vi "Main.vi"() -> ()   [LabVIEW 2017]
uses:
  CTL/REF Channel Select.ctl
  D:/test/PDLSTS/LV_PDL_Sample/DLL/STSProcess.dll
  DLL/STSProcess.dll
  CTL/Address Cluster.ctl
  D:/test/PDLSTS/LV_PDL_Sample/DLL/InstrumentDLL.dll
  DLL/InstrumentDLL.dll
  <vilib>/Utility/miscctls.llb/LVStringsAndValuesArrayTypeDef_DBL.ctl
panel:
  in  "btnsavecalil":bool
  in  "txtsaverange":i32=1 caption="Range"
  in  "chksavemu":bool
  in  "chk2scan":bool
  in  "PDLSTS":refnum<k24>
  in  "btnzeroing":bool
  in  "btnreadref_data":bool
  in  "btnsaveRawdata":bool
  in  "btnsaveref_rawdata":bool
  in  "chkeach_ch":bool
  in  "btnmeas":bool
  in  "btnset":bool
  in  "Range1":bool
  in  "REF Channel Select":T1={"M1S0C1"=TRUE, "M1S0C2"=FALSE, "M1S0C3"=FALSE, "M1S0C4"=FALSE, "M1S1C1"=FALSE, "M1S1C2"=FALSE, "M1S1C3"=FALSE, "M1S1C4"=FALSE, "M1S2C1"=FALSE, "M1S2C2"=FALSE, "M1S2C3"=FALSE, "M1S2C4"=FALSE, "M1S3C1"=FALSE, "M1S3C2"=FALSE, "M1S3C3"=FALSE, "M1S3C4"=FALSE, "M1S4C1"=FALSE, "M1S4C2"=FALSE, "M1S4C3"=FALSE, "M1S4C4"=FALSE, "M2S0C1"=FALSE, "M2S0C2"=FALSE, "M2S0C3"=FALSE, "M2S0C4"=FALSE, "M2S1C1"=FALSE, "M2S1C2"=FALSE, "M2S1C3"=FALSE, "M2S1C4"=FALSE, "M2S2C1"=FALSE, "M2S2C2"=FALSE, "M2S2C3"=FALSE, "M2S2C4"=FALSE, "M2S3C1"=FALSE, "M2S3C2"=FALSE, "M2S3C3"=FALSE, "M2S3C4"=FALSE, "M2S4C1"=FALSE, "M2S4C2"=FALSE, "M2S4C3"=FALSE, "M2S4C4"=FALSE}
  in  "Range2":bool
  in  "Range3":bool
  in  "Range4":bool
  in  "Range5":bool
  in  "btnget_reference":bool
  in  "Address Cluster":T2={"SPU"=refnum, "MPM"=[], "Port_Count"=0.0, "MPM_Count"=0.0, "SPU_Resource"=[], "USB_Resource"=[], "MPM_Communicater"="", "MPM_Count"=0.0, "MPM_Address"=[], "MPM_Portnumber"=[], "SPU_DeviveID"="", "MPM_communcation_method"=[], "TSL_sweepstartwave"=0.0, "TSL_sweepstopwave"=0.0, "TSL_Address"="", "TSL_Communicater"="", "TSL"=refnum, "tsl_communcation_method"=3, "TSL_Portnumber"=0.0, "PCU"=refnum, "PCU_Communicater"="", "PCU_Address"="", "PCU_Portnumber"=0.0, "PCU_useing_internal_DAQ"=FALSE, "PCU_communcation_method"=0} {"PCU_communcation_method" items=["GPIB", "C232C", "TCPIP", "USB"]; "tsl_communcation_method" items=["GPIB", "C232C", "TCPIP", "USB"]; "MPM_communcation_method" items=["GPIB", "C232C", "TCPIP", "USB"]}
  in  "Active Sensors":bool[](array[boolean])
  out "Meas_rang":i32[](array[numeric])
  out "Flag_213":bool
  out "Flag_215":bool
  out "Mergedata_struct":refnum<k24>[](array[refnum])
  out "Meas_monitor_struct":refnum<k24>[](array[refnum])
  out "Ref_monitordata_struct":refnum<k24>[](array[refnum])
  out "Refdata_struct":refnum<k24>[](array[refnum])
  out "Data_struct":refnum<k24>[](array[refnum])
  in  "txtpower":dbl caption="TSL Power(dBm)"
  in  "cmbspeed":u16(ring) caption="SweepSpeed(nm/sec)" items=["1"=1, "5"=5, "10"=10, "20"=20, "40"=40, "50"=50, "80"=80, "100"=100]
  in  "txtstepwave":dbl=0.01 caption="WavelengthStep(nm)"
  in  "txtstopwave":dbl caption="StopWavelength(nm)"
  in  "txtstartwave":dbl caption="StartWavelength(nm)"
  # "Measurement ch"
  # "Measurement Range"
  # "PDL Calcurate"
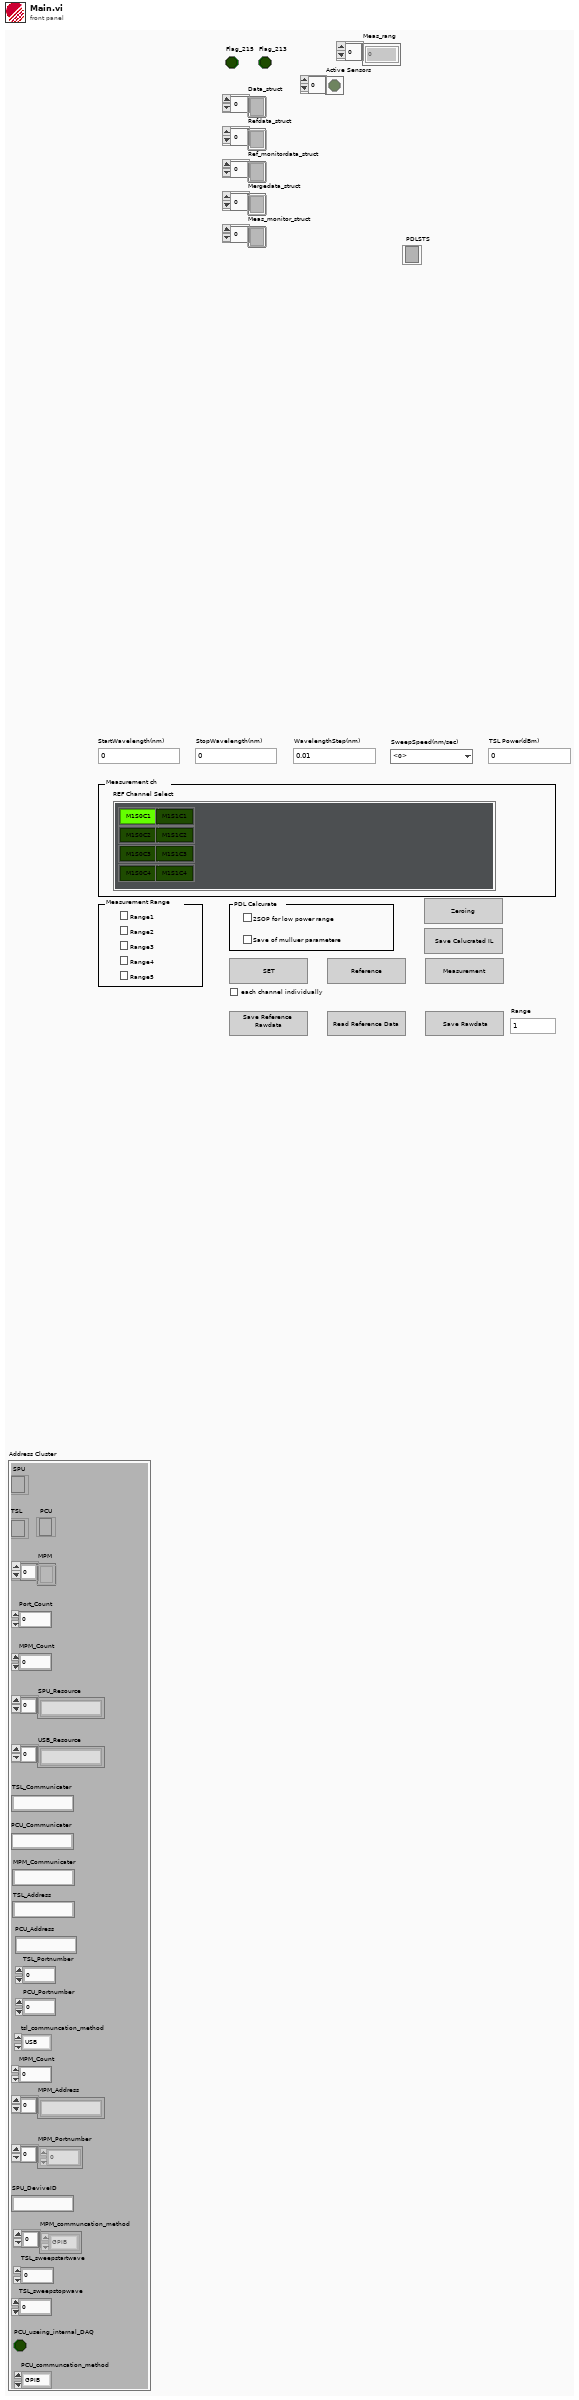
[diagram p1: front panel]
types:
  T1 = typedef "REF Channel Select.ctl" = cluster{"M1S0C1":bool, "M1S0C2":bool, "M1S0C3":bool, "M1S0C4":bool, "M1S1C1":bool, "M1S1C2":bool, "M1S1C3":bool, "M1S1C4":bool, "M1S2C1":bool, "M1S2C2":bool, "M1S2C3":bool, "M1S2C4":bool, "M1S3C1":bool, "M1S3C2":bool, "M1S3C3":bool, "M1S3C4":bool, "M1S4C1":bool, "M1S4C2":bool, "M1S4C3":bool, "M1S4C4":bool, "M2S0C1":bool, "M2S0C2":bool, "M2S0C3":bool, "M2S0C4":bool, "M2S1C1":bool, "M2S1C2":bool, "M2S1C3":bool, "M2S1C4":bool, "M2S2C1":bool, "M2S2C2":bool, "M2S2C3":bool, "M2S2C4":bool, "M2S3C1":bool, "M2S3C2":bool, "M2S3C3":bool, "M2S3C4":bool, "M2S4C1":bool, "M2S4C2":bool, "M2S4C3":bool, "M2S4C4":bool}
  T2 = typedef "Address Cluster.ctl" = cluster{"SPU":refnum<k24>, "MPM":refnum<k24>[], "Port_Count":dbl, "MPM_Count":dbl, "SPU_Resource":string[], "USB_Resource":string[], "MPM_Communicater":string, "MPM_Count":dbl, "MPM_Address":string[], "MPM_Portnumber":dbl[], "SPU_DeviveID":string, "MPM_communcation_method":i32[], "TSL_sweepstartwave":dbl, "TSL_sweepstopwave":dbl, "TSL_Address":string, "TSL_Communicater":string, "TSL":refnum<k24>, "tsl_communcation_method":i32, "TSL_Portnumber":dbl, "PCU":refnum<k24>, "PCU_Communicater":string, "PCU_Address":string, "PCU_Portnumber":dbl, "PCU_useing_internal_DAQ":bool, "PCU_communcation_method":i32}
  T3 = enum8{"Enabled", "Disabled", "Disabled and Grayed Out"}
  T4 = typedef "LVStringsAndValuesArrayTypeDef_DBL.ctl" = cluster{"String":string, "Value":dbl}[]
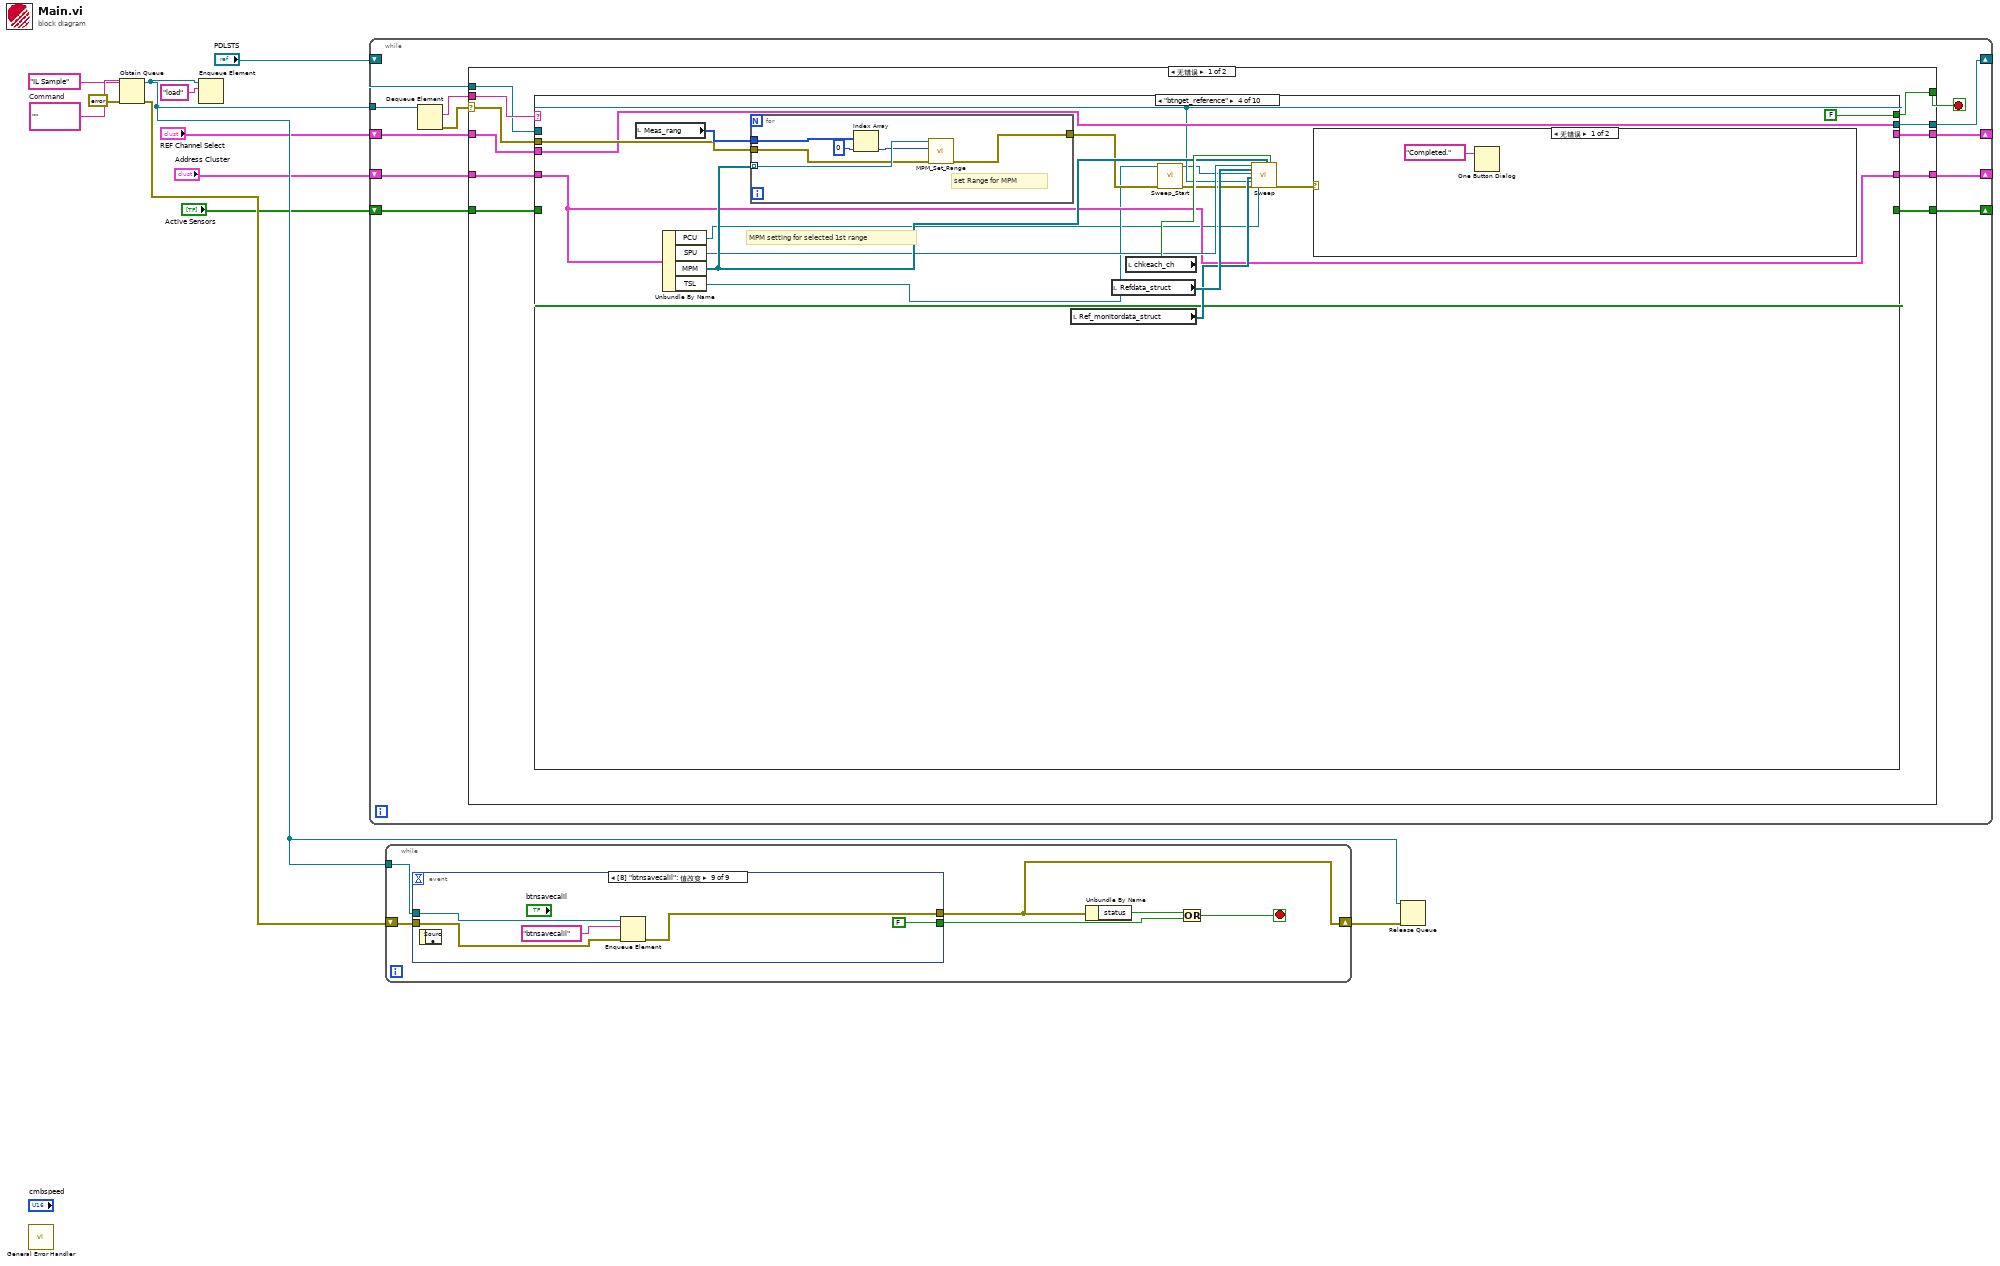
[diagram p0: block diagram]
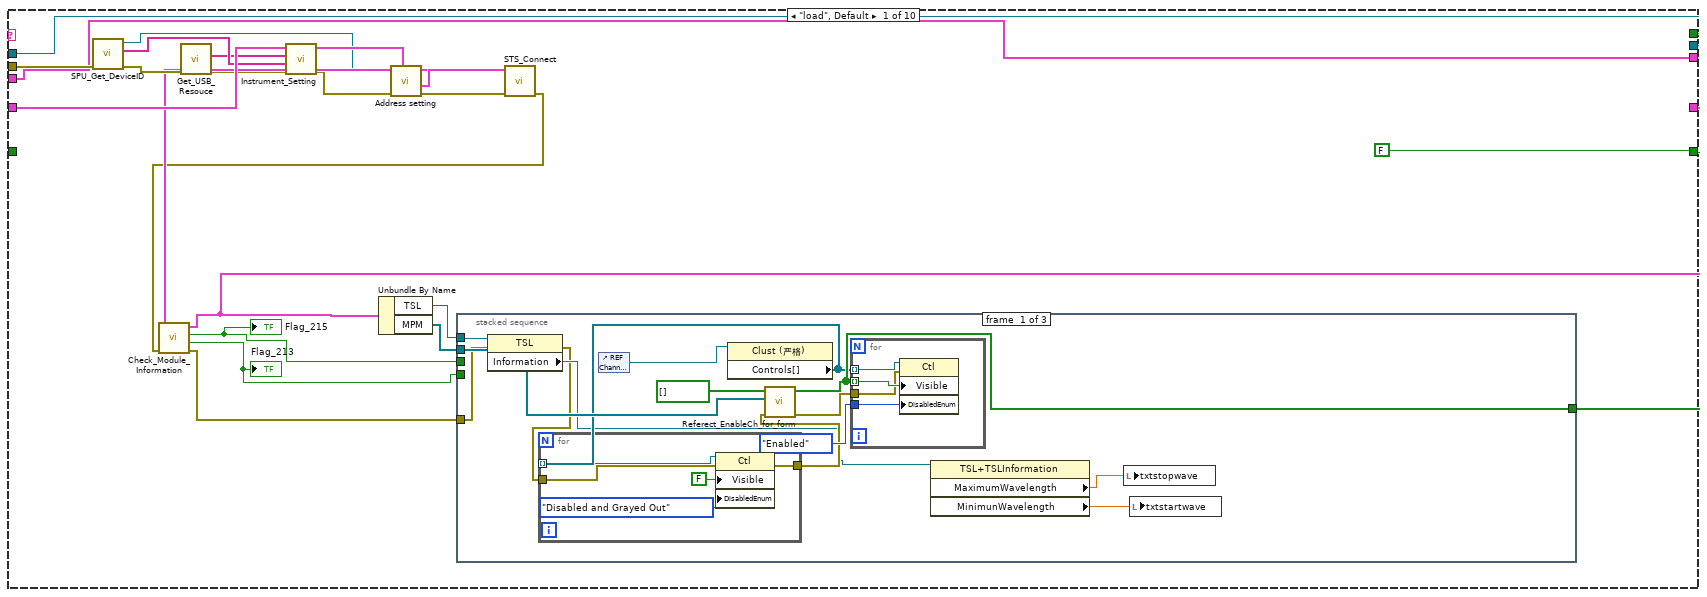
[diagram p2: hidden frame]
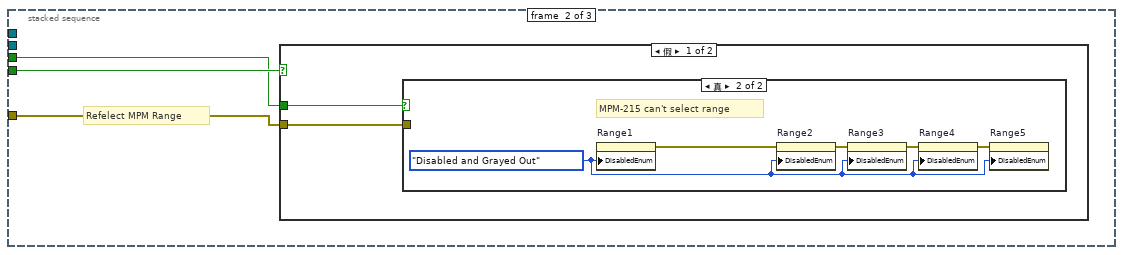
[diagram p3: hidden frame]
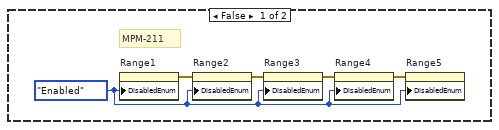
[diagram p4: hidden frame]
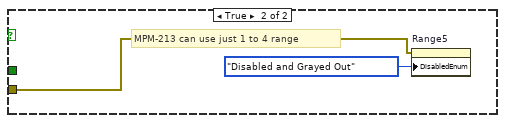
[diagram p5: hidden frame]
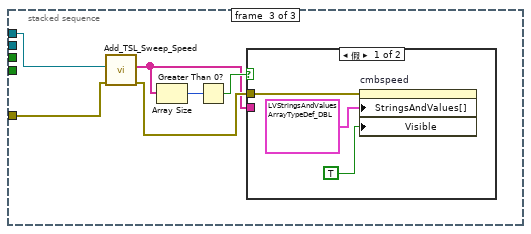
[diagram p6: hidden frame]
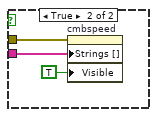
[diagram p7: hidden frame]
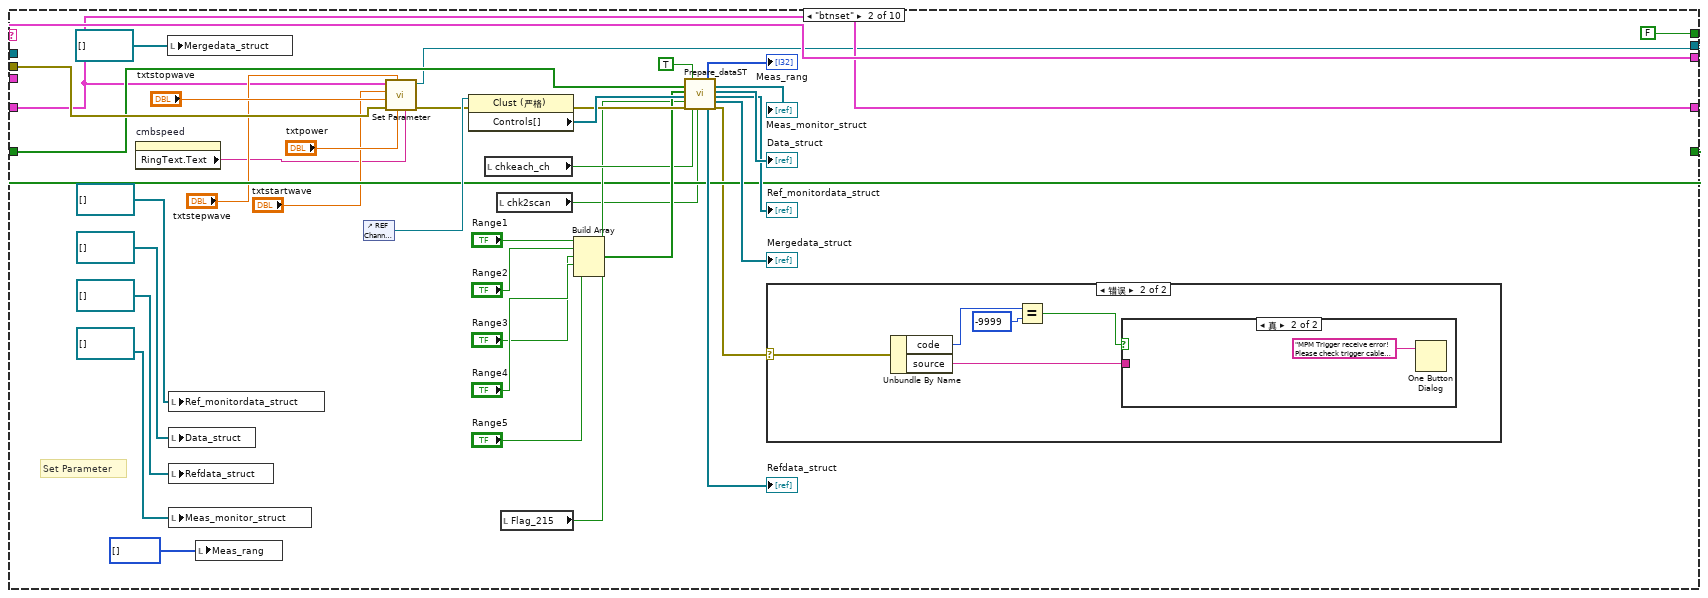
[diagram p8: hidden frame]
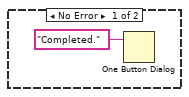
[diagram p9: hidden frame]
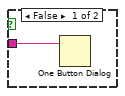
[diagram p10: hidden frame]
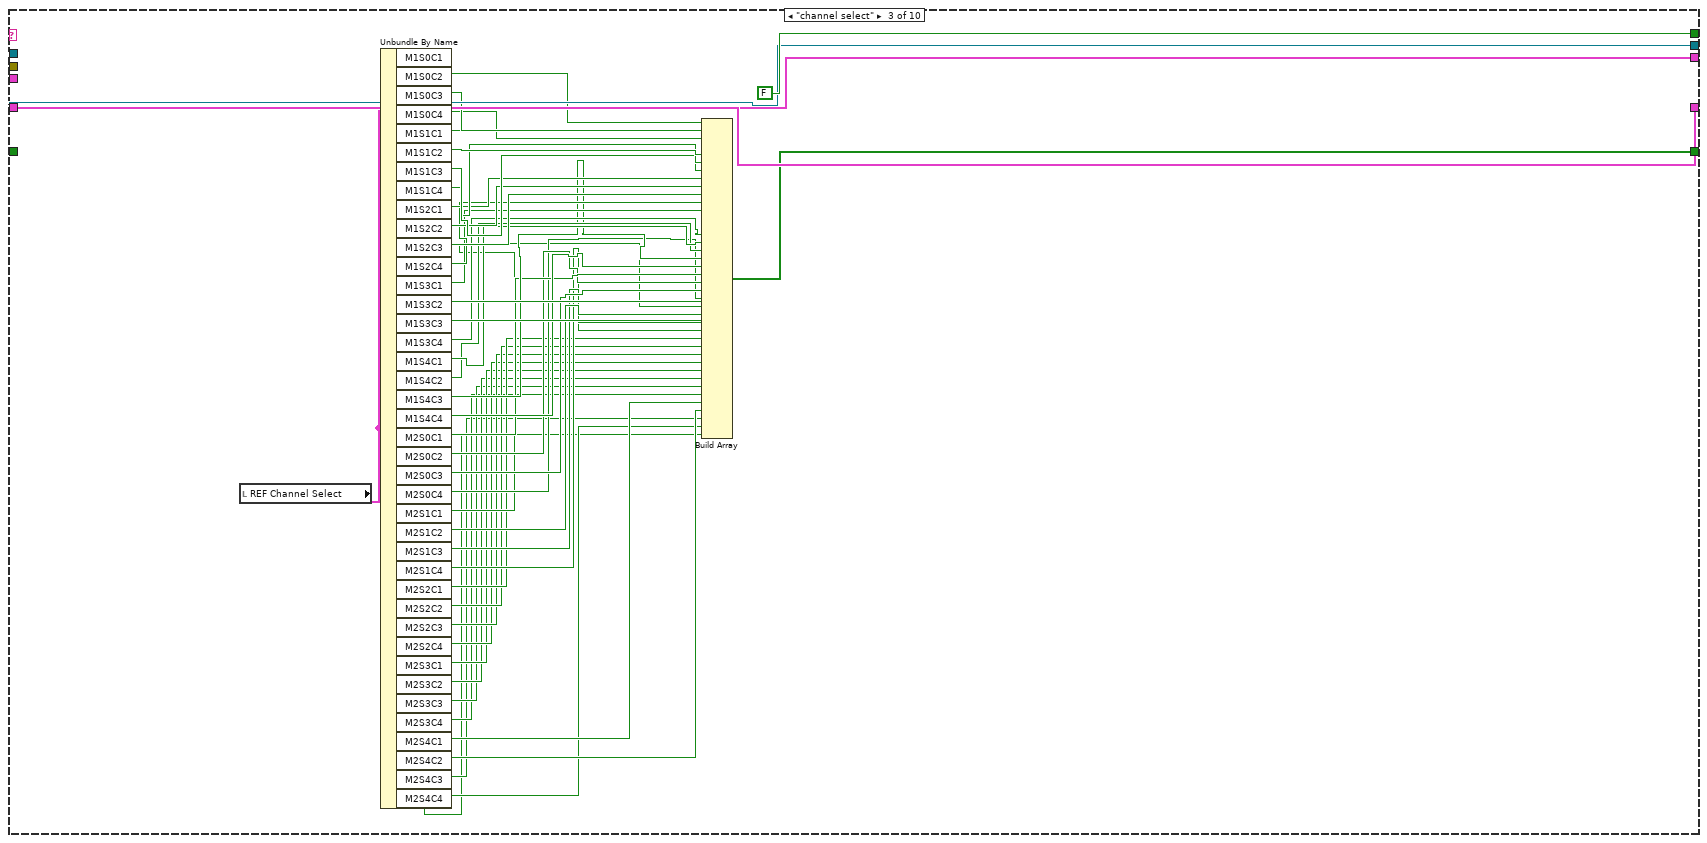
[diagram p11: hidden frame]
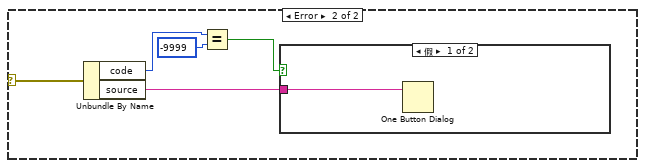
[diagram p12: hidden frame]
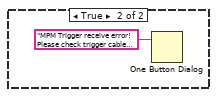
[diagram p13: hidden frame]
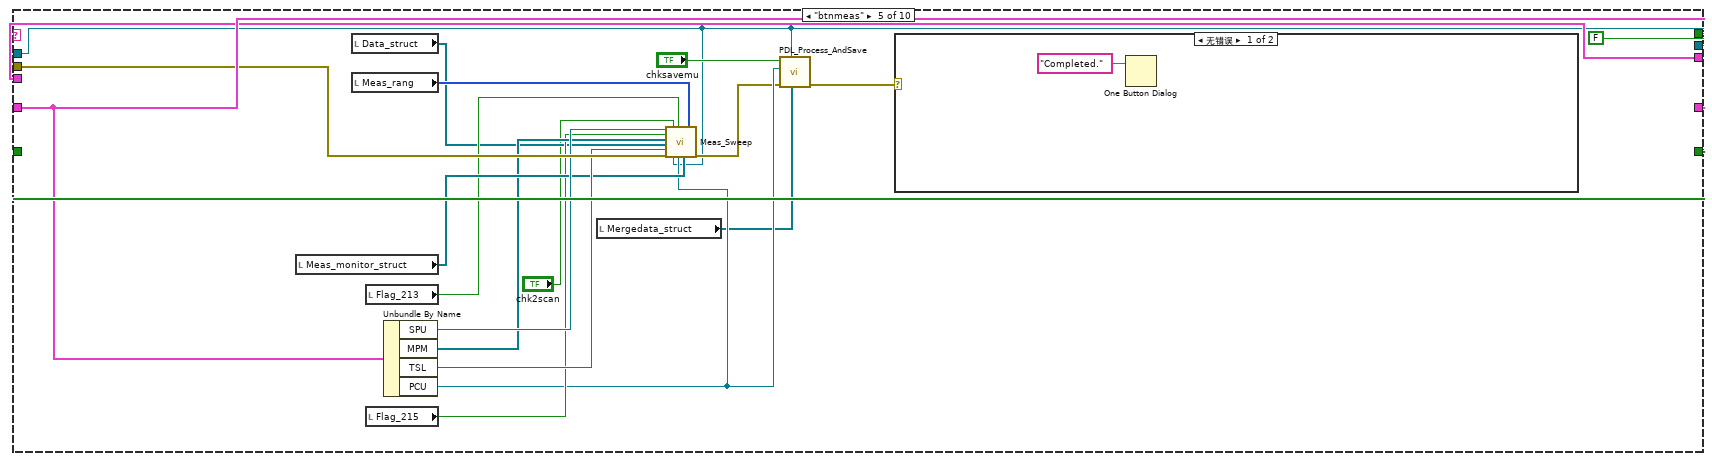
[diagram p14: hidden frame]
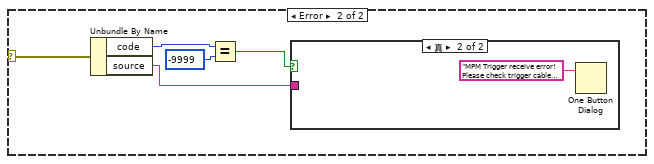
[diagram p15: hidden frame]
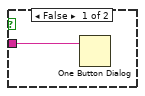
[diagram p16: hidden frame]
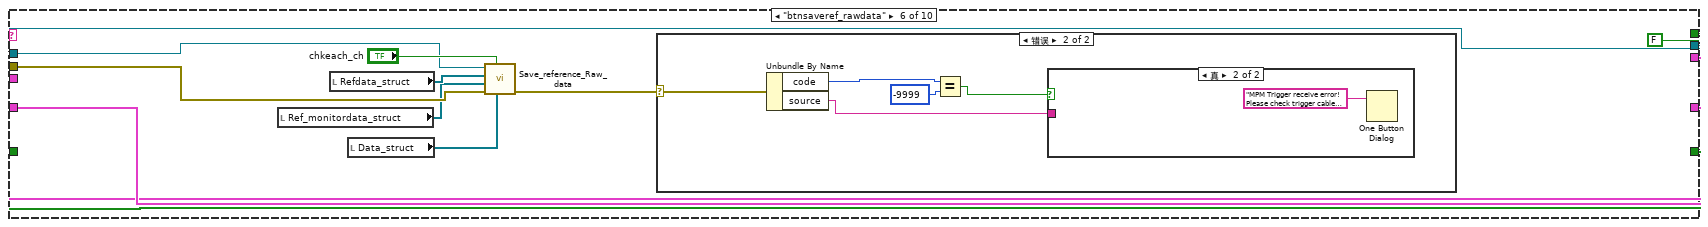
[diagram p17: hidden frame]
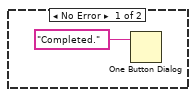
[diagram p18: hidden frame]
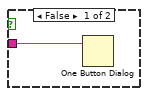
[diagram p19: hidden frame]
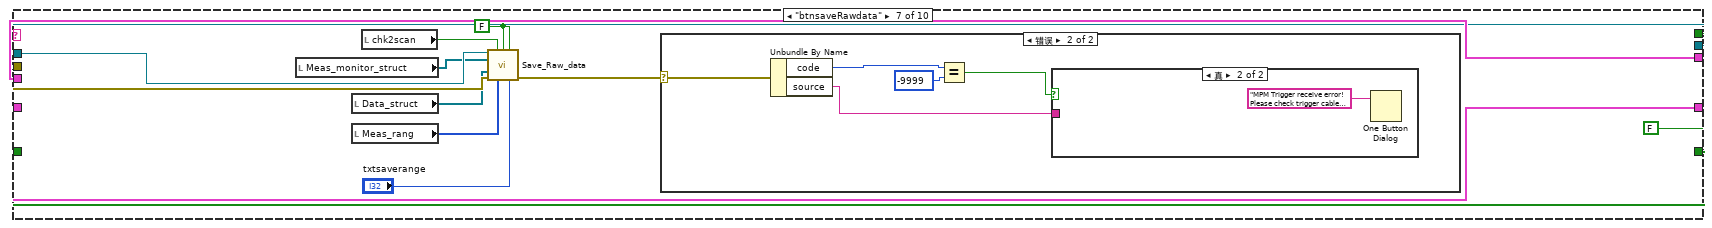
[diagram p20: hidden frame]
diagram:
  w11 = ""  # Command
  n1 = call <vilib>:"General Error Handler.vi"() -> ()  [unwired: 11 in, 5 out]
  n2 = Obtain Queue(name (unnamed)="IL Sample" ("名称（未命名）"), element data type=w11, error in (no error)=errorcluster {"status"=FALSE, "code"=0, "source"=""} ("错误输入（无错误）")) -> (queue out=w6:refnum<queue>, error out=w8:errorcluster)  [unwired: 2 in, 1 out]
  n3 = Enqueue Element(queue=w6, element="load" ("元素")) -> ()  [unwired: 2 in, 3 out]
  n4 = while {
    tunnel: w6 -> [w22]
    shift-right: [w18] -> _
    shift-left: "Address Cluster" -> [w19]
    shift-right: [w16] -> _
    shift-left: "PDLSTS" -> [w17]
    shift-right: [w15] -> _
    shift-left: "Active Sensors" -> [w14]
    shift-right: [w12] -> _
    shift-left: "REF Channel Select" -> [w13]
    stop <- w20 stop-if-true
    n5 = Dequeue Element(queue=w22) -> (element=w21:string, error out=w23:errorcluster)  [unwired: 2 in, 2 out]
    n6 = case shown="无错误" w23 {
      selector: w23 -> [w31 _]
      tunnel: w21 -> [w34 _]
      tunnel: [w33 TRUE] -> w20
      tunnel: w19 -> [w32 w356]
      tunnel: [w26 w356] -> w18
      tunnel: w17 -> [w30 w354]
      tunnel: [w29 w354] -> w16
      tunnel: [w28 w355] -> w15
      tunnel: w14 -> [w27 w355]
      tunnel: w13 -> [w25 w353]
      tunnel: [w24 w353] -> w12
      frame No Error {
        n7 = case shown="\"btnget_reference\"" w34 {
          tunnel: [FALSE FALSE FALSE FALSE FALSE FALSE FALSE FALSE FALSE FALSE] -> w33
          tunnel: w32 -> [w57 w113 w199 w209 w251 w270 w291 w304 w327 w342]
          tunnel: [w35 w113 w199 w209 w251 w270 w291 w304 w327 w342] -> w26
          tunnel: w31 -> [w56 w127 _ w217 w249 w268 w289 w302 w321 w340]
          tunnel: w30 -> [w43 _ w198 w204 w234 w264 w285 w305 w325 w338]
          tunnel: [w43 w112 w198 w204 w234 w264 w285 w305 w325 w338] -> w29
          tunnel: [w42 w126 w157 w210 w252 w271 w292 w308 w322 w341] -> w28
          tunnel: w27 -> [_ w126 _ w210 w252 w271 w292 w308 w322 w341]
          tunnel: w25 -> [w37 w125 _ w207 w248 w267 w288 w306 w328 w343]
          tunnel: [w37 w125 w156 w207 w248 w267 w288 w306 w328 w343] -> w24
          frame "load", Default {
            n8 = call "SPU_Get_DeviceID.vi"("错误输入（无错误）"=w56) -> ("error IO"=w53:errorcluster, "id"=w54:string[], "引用输出"=w48:refnum<k24>)  [unwired: 7 in]
            n9 = call "Get_USB_Resouce.vi"("error in (no error)"=w53) -> ("error out"=w47:errorcluster, "Get_USB_Resouce"=w52:string[])  [unwired: 8 in, 1 out]
            n10 = call "Instrument_Setting.vi"(8:w47, "id"=w54, "Get_USB_Resouce"=w52, "Address Cluster"=w57) -> ("错误输出"=w46:errorcluster, "Address Cluster out"=w51:T2)  [unwired: 6 in]
            n11 = call "Address setting.vi"("Address Cluster out输入"=w51, "错误输入（无错误）"=w46, "SPU in"=w48) -> ("error out"=w45:errorcluster, "Address Cluster out输出"=w50:T2)  [unwired: 7 in]
            n12 = call "STS_Connect.vi"("error in"=w45, "Address Cluster out输入"=w50) -> ("error out"=w44:errorcluster, "Address Cluster out"=w49:T2)  [unwired: 8 in]
            n13 = call "Check_Module_Information.vi"("Address Cluster"=w49, "错误输入（无错误）"=w44) -> ("Address Cluster out"=w35:T2, "Flag_215"=w40:bool, "Flag_213"=w41:bool, "error out"=w39:errorcluster)  [unwired: 5 in]
            "Flag_215" <- w40
            "Flag_213" <- w41
            n14 = Unbundle By Name(w35) -> ("TSL"=w38:refnum<k24>, "MPM"=w36:refnum<k24>[])
            n15 = stacked-sequence {
              tunnel: w36 -> [w71 _ _]
              tunnel: [w66 _ _] -> w42
              tunnel: w41 -> [_ w83 _]
              tunnel: w40 -> [_ w82 _]
              tunnel: w39 -> [w60 w81 w102]
              tunnel: w38 -> [w63 _ w103]
              frame #0 {
                n16 = property on="属性节点" class="TSL"(reference=w63, error in=w60) -> (error out=w58:errorcluster, "Information"=w59:refnum<k24>)  [unwired: 1 out]
                n17 = control-ref of="REF Channel Select"() -> (w69:refnum<vi>)
                n18 = property on="Property Node" class="Clust (严格)"(reference=w69) -> ("Controls[]"=w65:refnum<vi>[])  [unwired: 1 in, 2 out]
                n19 = for {
                  tunnel: w65 -> [w76] mode=indexing
                  tunnel: w58 -> [w73]
                  tunnel: [w72] -> w64
                  n20 = property on="Property Node" class="Ctl"(reference=w76, error in=w73, "Visible"=FALSE ("可见"), "DisabledEnum"=T3."Disabled and Grayed Out" ("禁用")) -> (error out=w72:errorcluster)  [unwired: 1 out]
                }
                n21 = call "Referect_EnableCh_for_form.vi"("错误输入（无错误）"=w64, "MPM"=w71, "数组输入"=bool[] []) -> ("error IO"=w67:errorcluster, "数组输出"=w66:bool[])  [unwired: 7 in]
                n22 = for {
                  tunnel: w65 -> [w80] mode=indexing
                  tunnel: w66 -> [w79] mode=indexing
                  tunnel: T3."Enabled" ("禁用") -> [w78]
                  tunnel: w67 -> [w77]
                  n23 = property on="Property Node" class="Ctl"(reference=w80, error in=w77, "Visible"=w79, "DisabledEnum"=w78) -> ()  [unwired: 2 out]
                }
                n24 = property on="属性节点" class="TSL+TSLInformation"(reference=w59) -> ("MaximumWavelength"=w61:dbl, "MinimunWavelength"=w62:dbl)  [unwired: 1 in, 2 out]
                n25 = local write "txtstopwave"(w61) -> ()
                n26 = local write "txtstartwave"(w62) -> ()
              }
              frame #1 {
                # "Refelect MPM Range"
                n27 = case shown="假" w83 {
                  tunnel: w82 -> [w85 _]
                  tunnel: w81 -> [w84 w96]
                  frame False {
                    n28 = case shown="真" w85 {
                      tunnel: w84 -> [_ _]
                      frame False {
                        w86 = T3."Enabled" ("禁用")
                        # "MPM-211"
                        n29 = property on="Range1" class="Bool (严格)"("DisabledEnum"=w86) -> (error out=w90:errorcluster)  [unwired: 2 in, 1 out]
                        n30 = property on="Range2" class="Bool (严格)"(error in=w90, "DisabledEnum"=w86) -> (error out=w89:errorcluster)  [unwired: 1 in, 1 out]
                        n31 = property on="Range3" class="Bool (严格)"(error in=w89, "DisabledEnum"=w86) -> (error out=w88:errorcluster)  [unwired: 1 in, 1 out]
                        n32 = property on="Range4" class="Bool (严格)"(error in=w88, "DisabledEnum"=w86) -> (error out=w87:errorcluster)  [unwired: 1 in, 1 out]
                        n33 = property on="Range5" class="Bool (严格)"(error in=w87, "DisabledEnum"=w86) -> ()  [unwired: 1 in, 2 out]
                      }
                      frame True {
                        w91 = T3."Disabled and Grayed Out" ("禁用")
                        # "MPM-215 can't select range"
                        n34 = property on="Range1" class="Bool (严格)"("DisabledEnum"=w91) -> (error out=w95:errorcluster)  [unwired: 2 in, 1 out]
                        n35 = property on="Range2" class="Bool (严格)"(error in=w95, "DisabledEnum"=w91) -> (error out=w94:errorcluster)  [unwired: 1 in, 1 out]
                        n36 = property on="Range3" class="Bool (严格)"(error in=w94, "DisabledEnum"=w91) -> (error out=w93:errorcluster)  [unwired: 1 in, 1 out]
                        n37 = property on="Range4" class="Bool (严格)"(error in=w93, "DisabledEnum"=w91) -> (error out=w92:errorcluster)  [unwired: 1 in, 1 out]
                        n38 = property on="Range5" class="Bool (严格)"(error in=w92, "DisabledEnum"=w91) -> ()  [unwired: 1 in, 2 out]
                      }
                    }
                  }
                  frame True {
                    # "MPM-213 can use just 1 to 4 range"
                    n39 = property on="Range5" class="Bool (严格)"(error in=w96, "DisabledEnum"=T3."Disabled and Grayed Out" ("禁用")) -> ()  [unwired: 1 in, 2 out]
                  }
                }
              }
              frame #2 {
                n40 = call "Add_TSL_Sweep_Speed.vi"("TSL"=w103, "error in (no error)"=w102) -> ("数组输出"=w98:string[], "error out"=w101:errorcluster)  [unwired: 7 in]
                n41 = Array Size(array=w98) -> (size(s)=w100:i32)
                n42 = Greater Than 0?(x=w100) -> (x > 0?=w99:bool)
                n43 = case shown="假" w99 {
                  tunnel: w101 -> [w105 w108]
                  tunnel: w98 -> [_ w107]
                  frame False {
                    n44 = property on="cmbspeed" class="Ring (严格)"(error in=w105, "StringsAndValues[]"=T4 [{"String"="1", "Value"=1.0}, {"String"="5", "Value"=5.0}, {"String"="10", "Value"=10.0}, {"String"="20", "Value"=20.0}, {"String"="40", "Value"=40.0}, {"String"="50", "Value"=50.0}, {"String"="80", "Value"=80.0}, {"String"="100", "Value"=100.0}] ("Strings And Values []"), "Visible"=TRUE ("可见")) -> ()  [unwired: 1 in, 2 out]
                  }
                  frame True {
                    n45 = property on="cmbspeed" class="Ring (严格)"(error in=w108, "Strings []"=w107, "Visible"=TRUE ("可见")) -> ()  [unwired: 1 in, 2 out]
                  }
                }
              }
            }
          }
          frame "btnset" {
            # "Set Parameter"
            n46 = property on="cmbspeed" class="Ring (严格)"() -> ("RingText.Text"=w115:string)  [unwired: 2 in, 2 out]
            n47 = local write "Mergedata_struct"(refnum<k24>[] [] ("Mergedata_struct")) -> ()
            n48 = local write "Ref_monitordata_struct"(refnum<k24>[] [] ("Ref_monitordata_struct")) -> ()
            n49 = local write "Data_struct"(refnum<k24>[] [] ("Data_struct")) -> ()
            n50 = local write "Refdata_struct"(refnum<k24>[] [] ("Refdata_struct")) -> ()
            n51 = local write "Meas_monitor_struct"(refnum<k24>[] [] ("Meas_monitor_struct")) -> ()
            n52 = local write "Meas_rang"(i32[] [] ("Meas_rang")) -> ()
            n53 = control-ref of="REF Channel Select"() -> (w146:refnum<vi>)
            n54 = call "Set Parameter.vi"("RingText.Text"=w115, "txtpower"="txtpower", "txtstepwave"="txtstepwave", "error in"=w127, "txtstopwave"="txtstopwave", "txtstartwave"="txtstartwave", "Address Cluster"=w113) -> ("error out"=w114:errorcluster, "PDLSTS"=w112:refnum<k24>)  [unwired: 3 in]
            n55 = property class="Clust (严格)"(reference=w146, error in=w114) -> (error out=w136:errorcluster, "Controls[]"=w137:refnum<vi>[])  [unwired: 1 out]
            n56 = local read "chkeach_ch"() -> (w134:bool)
            n57 = local read "chk2scan"() -> (w110:bool)
            n58 = local read "Flag_215"() -> (w133:bool)
            n59 = Build Array("Range1", "Range2", "Range3", "Range4", "Range5") -> (w135:bool[])
            n60 = call "Prepare_dataST.vi"("Active Sensors"=w126, "ranges"=w135, "Controls[]"=w137, "Flag_215"=w133, "error in"=w136, "struct"=TRUE, "chkeach_ch"=w134, "chk2scan"=w110) -> ("Meas_rang"=→"Meas_rang":i32[], "Refdata_struct"=→"Refdata_struct":refnum<k24>[], "Meas_monitor_struct"=→"Meas_monitor_struct":refnum<k24>[], "Data_struct"=→"Data_struct":refnum<k24>[], "Ref_monitordata_struct"=→"Ref_monitordata_struct":refnum<k24>[], "Mergedata_struct"=→"Mergedata_struct":refnum<k24>[], "error out"=w111:errorcluster)  [unwired: 5 in]
            n61 = case shown="错误" w111 {
              selector: w111 -> [_ w153]
              frame No Error {
                n62 = One Button Dialog(message="Completed." ("消息")) -> ()  [unwired: 1 in, 1 out]
              }
              frame Error {
                n63 = Unbundle By Name(w153) -> ("code"=w152:i32, "source"=w149:string)
                n64 = Equal?(x=w152, y=-9999) -> (x = y?=w150:bool)
                n65 = case shown="真" w150 {
                  tunnel: w149 -> [w154 _]
                  frame False {
                    n66 = One Button Dialog(message=w154) -> ()  [unwired: 1 in, 1 out]
                  }
                  frame True {
                    n67 = One Button Dialog(message="MPM Trigger receive error! Please check trigger cable connection." ("消息")) -> ()  [unwired: 1 in, 1 out]
                  }
                }
              }
            }
          }
          frame "channel select" {
            n68 = local read "REF Channel Select"() -> (w156:T1)
            n69 = Unbundle By Name(w156) -> ("M1S0C1"=w197:bool, "M1S0C2"=w196:bool, "M1S0C3"=w195:bool, "M1S0C4"=w194:bool, "M1S1C1"=w193:bool, "M1S1C2"=w192:bool, "M1S1C3"=w191:bool, "M1S1C4"=w190:bool, "M1S2C1"=w189:bool, "M1S2C2"=w188:bool, "M1S2C3"=w187:bool, "M1S2C4"=w186:bool, "M1S3C1"=w185:bool, "M1S3C2"=w184:bool, "M1S3C3"=w183:bool, "M1S3C4"=w182:bool, "M1S4C1"=w181:bool, "M1S4C2"=w180:bool, "M1S4C3"=w179:bool, "M1S4C4"=w178:bool, "M2S0C1"=w177:bool, "M2S0C2"=w176:bool, "M2S0C3"=w175:bool, "M2S0C4"=w174:bool, "M2S1C1"=w173:bool, "M2S1C2"=w172:bool, "M2S1C3"=w171:bool, "M2S1C4"=w170:bool, "M2S2C1"=w169:bool, "M2S2C2"=w168:bool, "M2S2C3"=w167:bool, "M2S2C4"=w166:bool, "M2S3C1"=w165:bool, "M2S3C2"=w164:bool, "M2S3C3"=w163:bool, "M2S3C4"=w162:bool, "M2S4C1"=w161:bool, "M2S4C2"=w160:bool, "M2S4C3"=w159:bool, "M2S4C4"=w158:bool)
            n70 = Build Array(w197, w196, w195, w194, w193, w192, w191, w190, w189, w188, w187, w186, w185, w184, w183, w182, w181, w180, w179, w178, w177, w176, w175, w174, w173, w172, w171, w170, w169, w168, w167, w166, w165, w164, w163, w162, w161, w160, w159, w158) -> (w157:bool[])
          }
          frame "btnget_reference" {
            # "MPM setting for selected 1st range"
            n71 = local read "Meas_rang"() -> (w218:i32[])
            n72 = Unbundle By Name(w209) -> ("PCU"=w202:refnum<k24>, "SPU"=w214:refnum<k24>, "MPM"=w215:refnum<k24>[], "TSL"=w203:refnum<k24>)
            n73 = for {
              tunnel: w215 -> [w232] mode=indexing
              tunnel: w218 -> [w231]
              tunnel: w217 -> [w228]
              tunnel: [w227] -> w206
              # "set Range for MPM"
              n74 = Index Array(array=w231, index=0 ("索引")) -> (element=w229:i32)
              n75 = call "MPM_Set_Range.vi"("error in (no error)"=w228, "Range All"=w229, ".NET Reference in"=w232) -> ("error out"=w227:errorcluster)  [unwired: 7 in, 1 out]
            }
            n76 = local read "Ref_monitordata_struct"() -> (w211:refnum<k24>[])
            n77 = local read "Refdata_struct"() -> (w212:refnum<k24>[])
            n78 = local read "chkeach_ch"() -> (w216:bool)
            n79 = call "Sweep_Start.vi"("error in (no error)"=w206, ".NET Reference in"=w203) -> ("error out"=w205:errorcluster, "Reference out"=w201:refnum<k24>)  [unwired: 8 in]
            n80 = call "Sweep.vi"("SPU"=w214, "Refdata_struct"=w212, "TSL"=w201, "Ref_monitordata_struct"=w211, "PDLSTS"=w204, "错误输入（无错误）"=w205, "PCU"=w202, "MPM"=w215, "chkeach_ch"=w216) -> ("错误输出"=w213:errorcluster)  [unwired: 10 in]
            n81 = case shown="无错误" w213 {
              selector: w213 -> [_ w224]
              frame No Error {
                n82 = One Button Dialog(message="Completed." ("消息")) -> ()  [unwired: 1 in, 1 out]
              }
              frame Error {
                n83 = Unbundle By Name(w224) -> ("code"=w223:i32, "source"=w220:string)
                n84 = Equal?(x=w223, y=-9999) -> (x = y?=w221:bool)
                n85 = case shown="假" w221 {
                  tunnel: w220 -> [w225 _]
                  frame False {
                    n86 = One Button Dialog(message=w225) -> ()  [unwired: 1 in, 1 out]
                  }
                  frame True {
                    n87 = One Button Dialog(message="MPM Trigger receive error! Please check trigger cable connection." ("消息")) -> ()  [unwired: 1 in, 1 out]
                  }
                }
              }
            }
          }
          frame "btnmeas" {
            n88 = local read "Meas_monitor_struct"() -> (w244:refnum<k24>[])
            n89 = local read "Data_struct"() -> (w240:refnum<k24>[])
            n90 = local read "Meas_rang"() -> (w246:i32[])
            n91 = local read "Flag_213"() -> (w241:bool)
            n92 = local read "Flag_215"() -> (w242:bool)
            n93 = Unbundle By Name(w251) -> ("SPU"=w245:refnum<k24>, "MPM"=w243:refnum<k24>[], "TSL"=w247:refnum<k24>, "PCU"=w238:refnum<k24>)
            n94 = local read "Mergedata_struct"() -> (w235:refnum<k24>[])
            n95 = call "Meas_Sweep.vi"("SPU"=w245, "Flag_215"=w242, "MPM"=w243, "Data_struct"=w240, "TSL"=w247, "错误输入（无错误）"=w249, "chk2scan"="chk2scan", "PDLSTS"=w234, "Flag_213"=w241, "PCU"=w238, "Meas_monitor_struct"=w244, "Meas_rang"=w246) -> ("错误输出"=w236:errorcluster)  [unwired: 7 in]
            n96 = call "PDL_Process_AndSave.vi"("Mergedata_struct"=w235, "PDLSTS"=w234, "错误输入（无错误）"=w236, "PCU"=w238, "chksavemu"="chksavemu") -> ("错误输出"=w233:errorcluster)  [unwired: 6 in]
            n97 = case shown="无错误" w233 {
              selector: w233 -> [_ w258]
              frame No Error {
                n98 = One Button Dialog(message="Completed." ("消息")) -> ()  [unwired: 1 in, 1 out]
              }
              frame Error {
                n99 = Unbundle By Name(w258) -> ("code"=w257:i32, "source"=w254:string)
                n100 = Equal?(x=w257, y=-9999) -> (x = y?=w255:bool)
                n101 = case shown="真" w255 {
                  tunnel: w254 -> [w259 _]
                  frame False {
                    n102 = One Button Dialog(message=w259) -> ()  [unwired: 1 in, 1 out]
                  }
                  frame True {
                    n103 = One Button Dialog(message="MPM Trigger receive error! Please check trigger cable connection." ("消息")) -> ()  [unwired: 1 in, 1 out]
                  }
                }
              }
            }
          }
          frame "btnsaveref_rawdata" {
            n104 = local read "Ref_monitordata_struct"() -> (w262:refnum<k24>[])
            n105 = local read "Refdata_struct"() -> (w263:refnum<k24>[])
            n106 = local read "Data_struct"() -> (w265:refnum<k24>[])
            n107 = call "Save_reference_Raw_data.vi"("Data_struct"=w265, "chkeach_ch"="chkeach_ch", "错误输入（无错误）"=w268, "Ref_monitordata_struct"=w262, "Refdata_struct"=w263, "PDLSTS"=w264) -> ("错误输出"=w261:errorcluster)  [unwired: 5 in]
            n108 = case shown="错误" w261 {
              selector: w261 -> [_ w277]
              frame No Error {
                n109 = One Button Dialog(message="Completed." ("消息")) -> ()  [unwired: 1 in, 1 out]
              }
              frame Error {
                n110 = Unbundle By Name(w277) -> ("code"=w276:i32, "source"=w273:string)
                n111 = Equal?(x=w276, y=-9999) -> (x = y?=w274:bool)
                n112 = case shown="真" w274 {
                  tunnel: w273 -> [w278 _]
                  frame False {
                    n113 = One Button Dialog(message=w278) -> ()  [unwired: 1 in, 1 out]
                  }
                  frame True {
                    n114 = One Button Dialog(message="MPM Trigger receive error! Please check trigger cable connection." ("消息")) -> ()  [unwired: 1 in, 1 out]
                  }
                }
              }
            }
          }
          frame "btnsaveRawdata" {
            w280 = FALSE ("first_rangeflag")
            n115 = local read "Meas_monitor_struct"() -> (w283:refnum<k24>[])
            n116 = local read "Data_struct"() -> (w284:refnum<k24>[])
            n117 = local read "Meas_rang"() -> (w287:i32[])
            n118 = local read "chk2scan"() -> (w282:bool)
            n119 = call "Save_Raw_data.vi"("PDLSTS"=w285, "chk2scan"=w282, "exist_flag"=w280, "first_rangeflag"=w280, "Meas_monitor_struct"=w283, "Data_struct"=w284, "错误输入（无错误）"=w289, "Meas_rang"=w287, "rangenumber"="txtsaverange") -> ("错误输出"=w286:errorcluster)  [unwired: 6 in]
            n120 = case shown="错误" w286 {
              selector: w286 -> [_ w298]
              frame No Error {
                n121 = One Button Dialog(message="Completed." ("消息")) -> ()  [unwired: 1 in, 1 out]
              }
              frame Error {
                n122 = Unbundle By Name(w298) -> ("code"=w297:i32, "source"=w294:string)
                n123 = Equal?(x=w297, y=-9999) -> (x = y?=w295:bool)
                n124 = case shown="真" w295 {
                  tunnel: w294 -> [w299 _]
                  frame False {
                    n125 = One Button Dialog(message=w299) -> ()  [unwired: 1 in, 1 out]
                  }
                  frame True {
                    n126 = One Button Dialog(message="MPM Trigger receive error! Please check trigger cable connection." ("消息")) -> ()  [unwired: 1 in, 1 out]
                  }
                }
              }
            }
          }
          frame "btnzeroing" {
            n127 = Unbundle By Name(w304) -> ("MPM"=w303:refnum<k24>[])
            n128 = for {
              tunnel: w303 -> [w311] mode=indexing
              tunnel: w302 -> [w310]
              tunnel: [w309] -> w301
              n129 = call "MPM_Zeroing.vi"("error in (no error)"=w310, ".NET Reference in"=w311) -> ("error out"=w309:errorcluster)  [unwired: 8 in, 1 out]
            }
            n130 = case shown="错误" w301 {
              selector: w301 -> [_ w317]
              frame No Error {
                n131 = One Button Dialog(message="Completed." ("消息")) -> ()  [unwired: 1 in, 1 out]
              }
              frame Error {
                n132 = Unbundle By Name(w317) -> ("code"=w316:i32, "source"=w313:string)
                n133 = Equal?(x=w316, y=-9999) -> (x = y?=w314:bool)
                n134 = case shown="假" w314 {
                  tunnel: w313 -> [w318 _]
                  frame False {
                    n135 = One Button Dialog(message=w318) -> ()  [unwired: 1 in, 1 out]
                  }
                  frame True {
                    n136 = One Button Dialog(message="MPM Trigger receive error! Please check trigger cable connection." ("消息")) -> ()  [unwired: 1 in, 1 out]
                  }
                }
              }
            }
          }
          frame "btnreadref_data" {
            n137 = Unbundle By Name(w327) -> ("TSL"=w326:refnum<k24>)
            n138 = local read "Data_struct"() -> (w323:refnum<k24>[])
            n139 = local read "chkeach_ch"() -> (w324:bool)
            n140 = call "Reference_Data_Read.vi"("Active Sensors"=w322, "chkeach_ch"=w324, "error in"=w321, "PDLSTS"=w325, "Data_struct"=w323, "TSL"=w326) -> ("error IO"=w320:errorcluster)  [unwired: 5 in]
            n141 = case shown="错误" w320 {
              selector: w320 -> [_ w335]
              frame No Error {
                n142 = One Button Dialog(message="Completed." ("消息")) -> ()  [unwired: 1 in, 1 out]
              }
              frame Error {
                n143 = Unbundle By Name(w335) -> ("code"=w334:i32, "source"=w331:string)
                n144 = Equal?(x=w334, y=-9999) -> (x = y?=w332:bool)
                n145 = case shown="假" w332 {
                  tunnel: w331 -> [w336 _]
                  frame False {
                    n146 = One Button Dialog(message=w336) -> ()  [unwired: 1 in, 1 out]
                  }
                  frame True {
                    n147 = One Button Dialog(message="MPM Trigger receive error! Please check trigger cable connection." ("消息")) -> ()  [unwired: 1 in, 1 out]
                  }
                }
              }
            }
          }
          frame "btnsavecalil" {
            n148 = call "Savecalil_data.vi"("错误输入（无错误）"=w340, "PDLSTS"=w338) -> ("错误输出"=w339:errorcluster)  [unwired: 9 in]
            n149 = case shown="无错误" w339 {
              selector: w339 -> [_ w350]
              frame No Error {
                n150 = One Button Dialog(message="Completed." ("消息")) -> ()  [unwired: 1 in, 1 out]
              }
              frame Error {
                n151 = Unbundle By Name(w350) -> ("code"=w349:i32, "source"=w346:string)
                n152 = Equal?(x=w349, y=-9999) -> (x = y?=w347:bool)
                n153 = case shown="假" w347 {
                  tunnel: w346 -> [w351 _]
                  frame False {
                    n154 = One Button Dialog(message=w351) -> ()  [unwired: 1 in, 1 out]
                  }
                  frame True {
                    n155 = One Button Dialog(message="MPM Trigger receive error! Please check trigger cable connection." ("消息")) -> ()  [unwired: 1 in, 1 out]
                  }
                }
              }
            }
          }
        }
      }
      frame Error {
      }
    }
  }
  n156 = while {
    tunnel: w6 -> [w362]
    shift-right: [w358] -> w7
    shift-left: w8 -> [w363]
    stop <- w360 stop-if-true
    n157 = event shown="[8] \"btnsavecalil\": 值改变" {
      selector: _ -> [_ _ _ _ _ _ _ _ _]
      dyn-events: _ -> [_ _ _ _ _ _ _ _ _]
      timeout: _ -> [_ _ _ _ _ _ _ _ _]
      tunnel: w363 -> [w366 w376 w381 w386 w391 w394 w399 w404 w409]
      tunnel: w362 -> [w367 w375 w380 w385 w390 w392 w397 w402 w407]
      tunnel: [w371 w374 w379 w384 w389 w393 w398 w403 w408] -> w358
      tunnel: [FALSE FALSE FALSE FALSE FALSE FALSE FALSE FALSE FALSE] -> w359
      event "btnset": Value Change {
        n158 = event-data() -> ()  [unwired: 1 in, 1 out]
        n159 = Enqueue Element(queue=w367, element="channel select" ("元素"), error in (no error)=w366) -> (queue out=w364:refnum<queue>, error out=w365:errorcluster)  [unwired: 1 in, 1 out]
        n160 = Enqueue Element(queue=w364, element="btnset" ("元素"), error in (no error)=w365) -> (error out=w371:errorcluster)  [unwired: 1 in, 2 out]
      }
      event "btnget_reference": Value Change {
        n161 = event-data() -> ()  [unwired: 1 in, 1 out]
        n162 = Enqueue Element(queue=w375, element="btnget_reference" ("元素"), error in (no error)=w376) -> (error out=w374:errorcluster)  [unwired: 1 in, 2 out]
      }
      event "btnmeas": Value Change {
        n163 = event-data() -> ()  [unwired: 1 in, 1 out]
        n164 = Enqueue Element(queue=w380, element="btnmeas" ("元素"), error in (no error)=w381) -> (error out=w379:errorcluster)  [unwired: 1 in, 2 out]
      }
      event "btnzeroing": Value Change {
        n165 = event-data() -> ()  [unwired: 1 in, 1 out]
        n166 = Enqueue Element(queue=w385, element="btnzeroing" ("元素"), error in (no error)=w386) -> (error out=w384:errorcluster)  [unwired: 1 in, 2 out]
      }
      event "btnsaveref_rawdata": Value Change {
        n167 = event-data() -> ()  [unwired: 1 in, 1 out]
        n168 = Enqueue Element(queue=w390, element="btnsaveref_rawdata" ("元素"), error in (no error)=w391) -> (error out=w389:errorcluster)  [unwired: 1 in, 2 out]
      }
      event Value Change {
        n169 = event-data() -> ()  [unwired: 1 in, 1 out]
        n170 = Enqueue Element(queue=w392, element="channel select" ("元素"), error in (no error)=w394) -> (error out=w393:errorcluster)  [unwired: 1 in, 2 out]
      }
      event "btnreadref_data": Value Change {
        n171 = event-data() -> ()  [unwired: 1 in, 1 out]
        n172 = Enqueue Element(queue=w397, element="btnreadref_data" ("元素"), error in (no error)=w399) -> (error out=w398:errorcluster)  [unwired: 1 in, 2 out]
      }
      event "btnsaveRawdata": Value Change {
        n173 = event-data() -> ()  [unwired: 1 in, 1 out]
        n174 = Enqueue Element(queue=w402, element="btnsaveRawdata" ("元素"), error in (no error)=w404) -> (error out=w403:errorcluster)  [unwired: 1 in, 2 out]
      }
      event "btnsavecalil": Value Change {
        n175 = event-data() -> ()  [unwired: 1 in, 1 out]
        n176 = Enqueue Element(queue=w407, element="btnsavecalil" ("元素"), error in (no error)=w409) -> (error out=w408:errorcluster)  [unwired: 1 in, 2 out]
      }
    }
    n177 = Unbundle By Name(w358) -> ("status"=w361:bool)
    n178 = Or(x=w361, y=w359) -> (x .or. y?=w360:bool)
  }
  n179 = Release Queue(queue=w6, error in (no error)=w7) -> ()  [unwired: 1 in, 3 out]
